vi "3-Bit Down Counter Controller(David Documentation).vi"(7 "Input":fxp<+,3,3>, 8 "Decrement?":bool, 9 "Load?":bool, 11 "Value":fxp<+,3,3>) -> (3 "Value+":fxp<+,3,3>)   [LabVIEW 2015]
doc: "This VI is going to count down depending on Load? input\nLoad? = True: load the Input Value.\nLoad? = False: counting down."
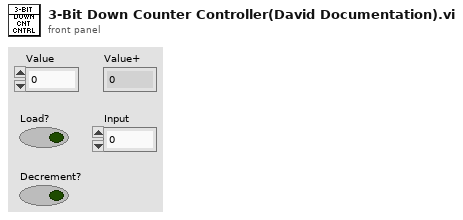
[diagram p1: front panel]
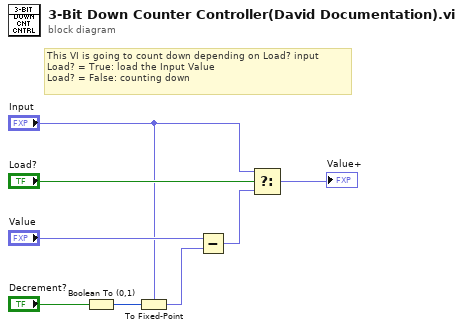
[diagram p0: block diagram]
diagram:
  # "This VI is going to count down depending on Load? input\nLoad? = True: load the Input Value\nLoad? = False: counting down"
  n1 = Boolean To (0,1)(Boolean="Decrement?") -> (0, 1=w3:i16)
  n2 = To Fixed-Point(fixed-point type="Input", number=w3) -> (fixed-point=w2:fxp<+,3,3>)
  n3 = Subtract(x="Value", y=w2) -> (x-y=w5:fxp<+,3,3>)
  n4 = Select(t="Input", s="Load?", f=w5) -> (s? t:f=→"Value+":fxp<+,3,3>)
